vi "CLD 4 Event Structure Time Out Front Panel - Solution.vi"() -> ()   [LabVIEW 2020]
doc: "CLD 4 exercise"
panel:
  in  "Decrement":bool
  out "Error Out":errorcluster
  in  "Error In":errorcluster
  out "Time Has Elapsed":bool
  out "Count":u32
  in  "Increment":bool
  in  "Stop VI":bool
  in  "Timeout Target (s)":dbl=2.0
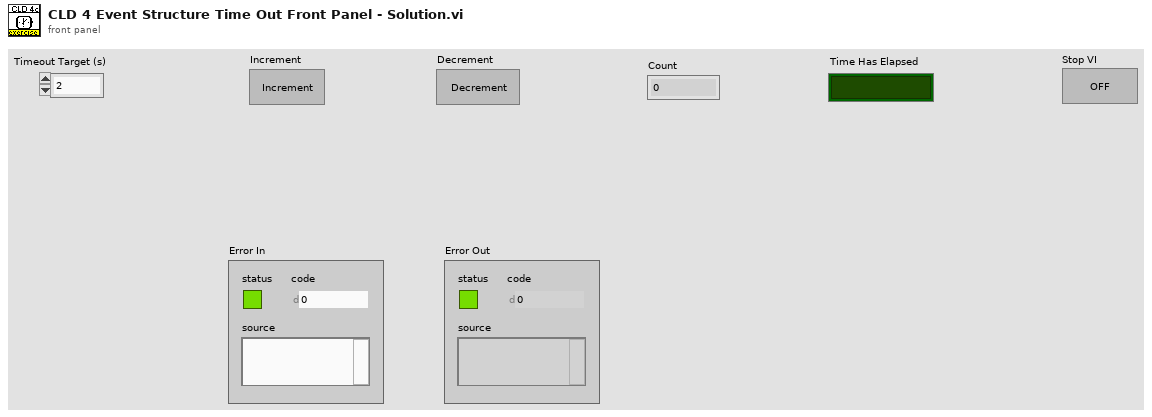
[diagram p1: front panel]
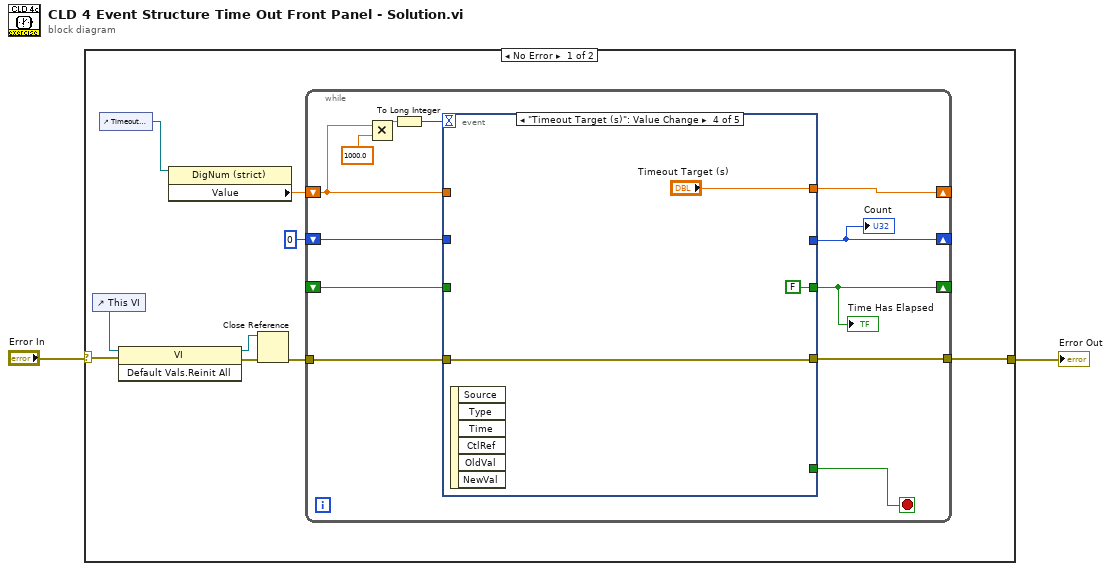
[diagram p0: block diagram]
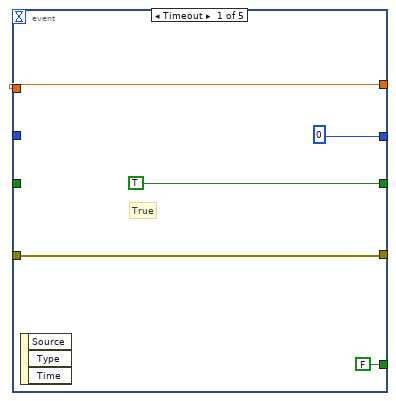
[diagram p2: hidden frame]
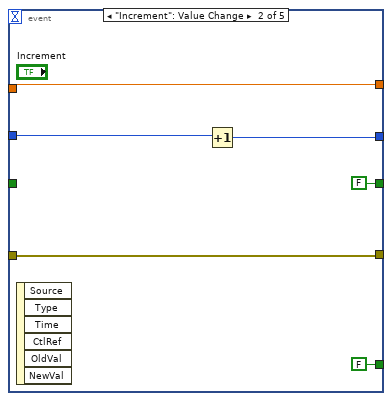
[diagram p3: hidden frame]
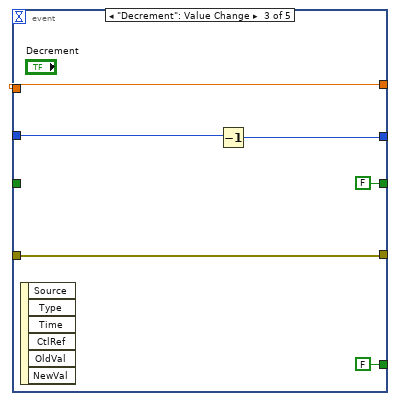
[diagram p4: hidden frame]
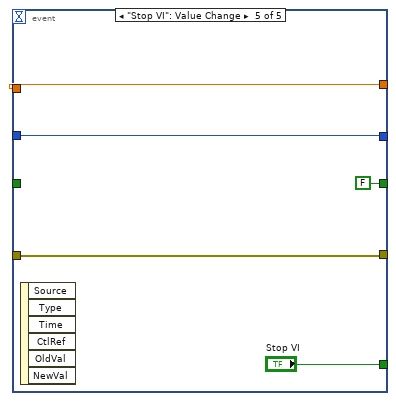
[diagram p5: hidden frame]
diagram:
  n1 = case shown="No Error" "Error In" {
    selector: "Error In" -> [w10 w49]
    tunnel: [w6 w49] -> w1
    frame No Error {
      n2 = control-ref of="This VI"() -> (w5:refnum<vi>)
      n3 = control-ref of="Timeout Target (s)"() -> (w4:refnum<vi>)
      n4 = invoke class="VI" method="Default Vals.Reinit All"(reference=w5, error in=w10) -> (reference out=w8:refnum<vi>, error out=w9:errorcluster)  [unwired: 1 in, 1 out]
      n5 = property class="DigNum (strict)"(reference=w4) -> ("Value"=w3:dbl)  [unwired: 1 in, 2 out]
      n6 = Close Reference(reference=w8, error in (no error)=w9) -> (error out=w7:errorcluster)
      n7 = while {
        shift-right: [w22] -> _
        shift-left: w3 -> [w16]
        shift-right: [w21] -> _
        shift-left: u32 0 -> [w20]
        shift-right: [w19] -> _
        shift-left: _ -> [w18]
        tunnel: w7 -> [w15]
        tunnel: [w14] -> w6
        stop <- w23 stop-if-true
        n8 = Multiply(x=w16, y=1000.0) -> (x*y=w13:dbl)
        n9 = To Long Integer(number=w13) -> (32bit integer=w12:i32)
        n10 = event shown="[3] \"Timeout Target (s)\": Value Change" {
          selector: _ -> [_ _ _ _ _]
          dyn-events: _ -> [_ _ _ _ _]
          timeout: w12 -> [_ _ _ _ _]
          tunnel: [FALSE ("Stop VI") FALSE ("Stop VI") FALSE ("Stop VI") _ "Stop VI"] -> w23
          tunnel: [w25 w30 w36 "Timeout Target (s)" w46] -> w22
          tunnel: [u32 0 w32 w38 _ w45] -> w21
          tunnel: w20 -> [_ w33 w39 _ w45]
          tunnel: [TRUE ("Time Has Elapsed") FALSE ("Time Has Elapsed") FALSE ("Time Has Elapsed") FALSE ("Time Has Elapsed") FALSE ("Time Has Elapsed")] -> w19
          tunnel: w18 -> [_ _ _ _ _]
          tunnel: w16 -> [w25 w30 w36 _ w46]
          tunnel: w15 -> [w24 w29 w35 w41 w44]
          tunnel: [w24 w29 w35 w41 w44] -> w14
          event Timeout {
            # "True"
            n11 = event-data() -> ()  [unwired: 1 in, 3 out]
          }
          event "Increment": Value Change {
            n12 = event-data() -> ()  [unwired: 1 in, 6 out]
            n13 = Increment(x=w33) -> (x+1=w32:u32)
          }
          event "Decrement": Value Change {
            n14 = event-data() -> ()  [unwired: 1 in, 6 out]
            n15 = Decrement(x=w39) -> (x-1=w38:u32)
          }
          event "Timeout Target (s)": Value Change {
            n16 = event-data() -> ()  [unwired: 1 in, 6 out]
          }
          event "Stop VI": Value Change {
            n17 = event-data() -> ()  [unwired: 1 in, 6 out]
          }
        }
        "Count" <- w21
        "Time Has Elapsed" <- w19
      }
    }
    frame Error {
    }
  }
  "Error Out" <- w1
